vi "Round_to_Digit.vi"(2 "Value to Round":dbl, 3 "Round to Value":dbl) -> (1 "Rounded Value":dbl)   [LabVIEW 2017]
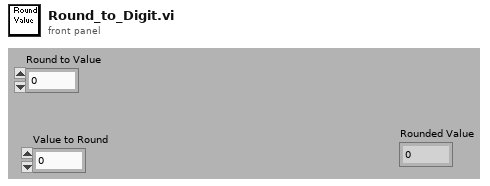
[diagram p1: front panel]
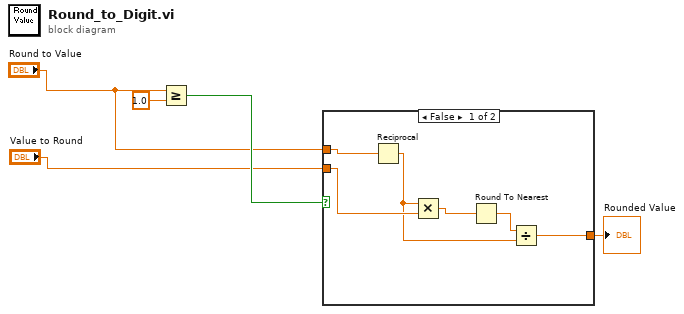
[diagram p0: block diagram]
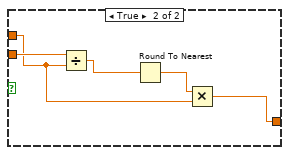
[diagram p2: hidden frame]
diagram:
  n1 = Greater Or Equal?(x="Round to Value", y=1.0) -> (x >= y?=w4:bool)
  n2 = case shown="False" w4 {
    tunnel: "Value to Round" -> [w10 w15]
    tunnel: "Round to Value" -> [w11 w12]
    tunnel: [w6 w16] -> w1
    frame False {
      n3 = Reciprocal(x=w11) -> (1/x=w7:dbl)
      n4 = Multiply(x=w7, y=w10) -> (x*y=w9:dbl)
      n5 = Round To Nearest(number=w9) -> (nearest integer value=w8:dbl)
      n6 = Divide(x=w8, y=w7) -> (x/y=w6:dbl)
    }
    frame True {
      n7 = Divide(x=w15, y=w12) -> (x/y=w14:dbl)
      n8 = Round To Nearest(number=w14) -> (nearest integer value=w13:dbl)
      n9 = Multiply(x=w13, y=w12) -> (x*y=w16:dbl)
    }
  }
  "Rounded Value" <- w1
